vi "GetWidth.vi"(8 "error in (no error)":errorcluster, 11 "Pen in":refnum<class "Pen.lvclass">) -> (0 "error out":errorcluster, 2 "Width":u16=1, 3 "Pen out":refnum<class "Pen.lvclass">)   [LabVIEW 2021, in "Picture2D.lvlib" / "Pen.lvclass"]
uses:
  Pen.lvclass
  Pen.lvclass/Pen.ctl
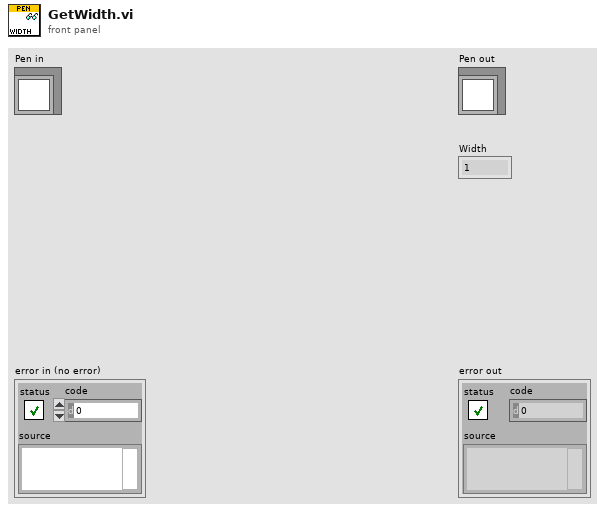
[diagram p1: front panel]
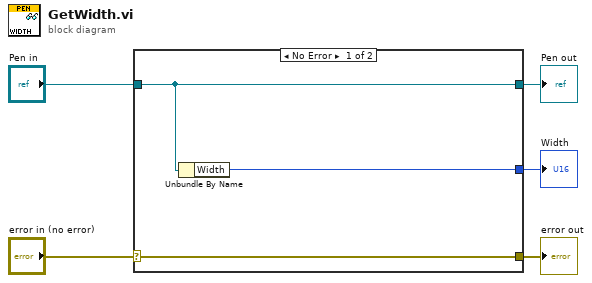
[diagram p0: block diagram]
diagram:
  n1 = case shown="No Error" "error in (no error)" {
    selector: "error in (no error)" -> [w8 w9]
    tunnel: [w8 w9] -> w4
    tunnel: [w7 w10] -> w2
    tunnel: "Pen in" -> [w7 w10]
    tunnel: [w6 _] -> w1
    frame No Error {
      n2 = Unbundle By Name(w7) -> ("Width"=w6:u16)
    }
    frame Error {
    }
  }
  "error out" <- w4
  "Pen out" <- w2
  "Width" <- w1
